vi "Set Window Position.vi"(7 "Module type":T1, 8 "error in (no error)":errorcluster, 11 "Vi reference":refnum<vi>) -> (0 "error out":errorcluster)   [LabVIEW 2021, in "Panther Dashboard.lvlib"]
uses:
  Panther Dashboard.lvlib
  Window Position--enum.ctl
  <vilib>/Utility/miscctls.llb/LVPointTypeDef.ctl
  <vilib>/Utility/miscctls.llb/LVRectTypeDef.ctl
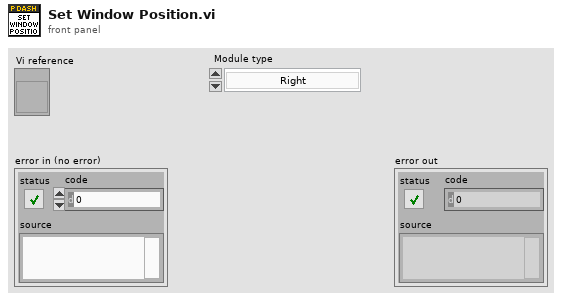
[diagram p1: front panel]
types:
  T1 = typedef "Panther Dashboard.lvlib/Window Position--enum.ctl" = enum16{"Right", "Left", "Center", "Max"}
  T2 = typedef "LVRectTypeDef.ctl" = cluster{"Left":i16, "Top":i16, "Right":i16, "Bottom":i16}
  T3 = typedef "LVPointTypeDef.ctl" = cluster{"Horizontal":i16, "Vertical":i16}
  T4 = enum32{"Invalid", "Standard", "Closed", "Hidden", "Minimized", "Maximized"}
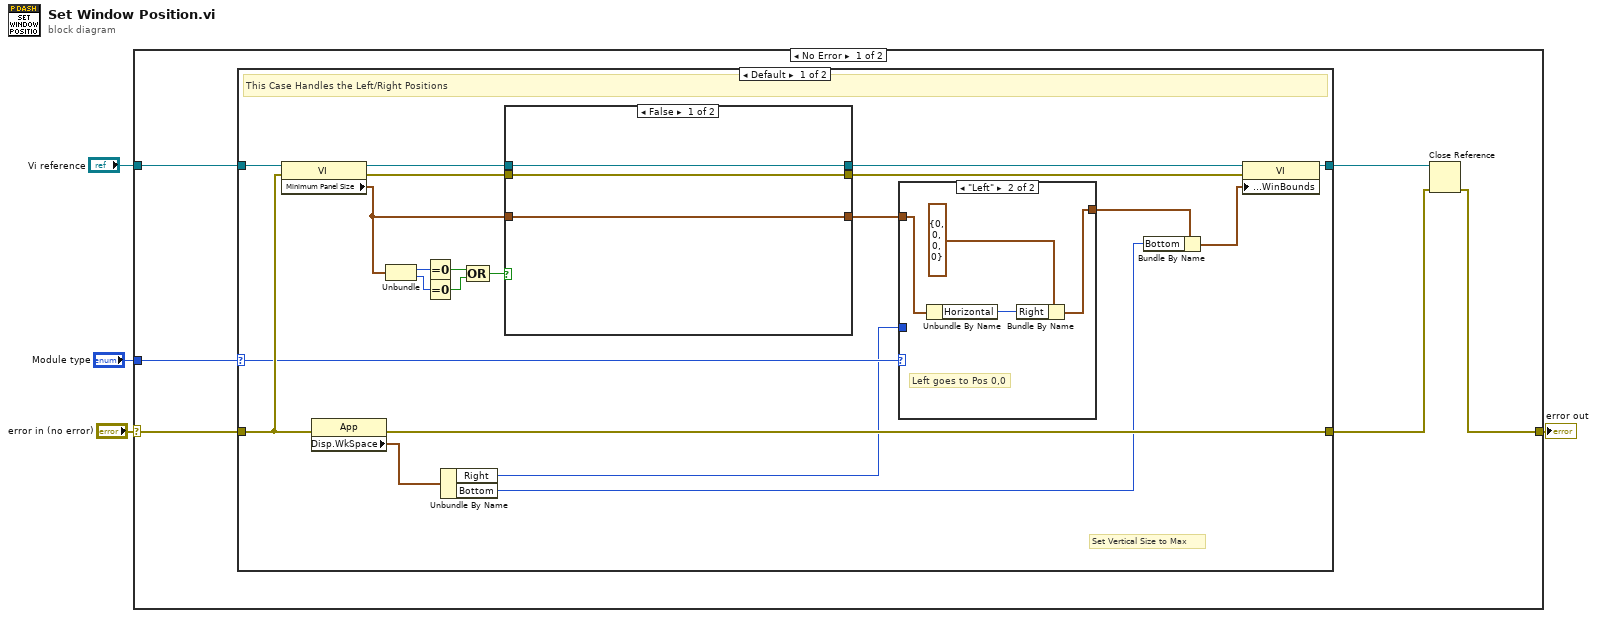
[diagram p0: block diagram]
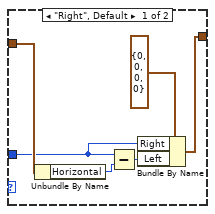
[diagram p2: hidden frame]
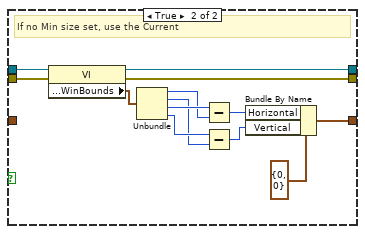
[diagram p3: hidden frame]
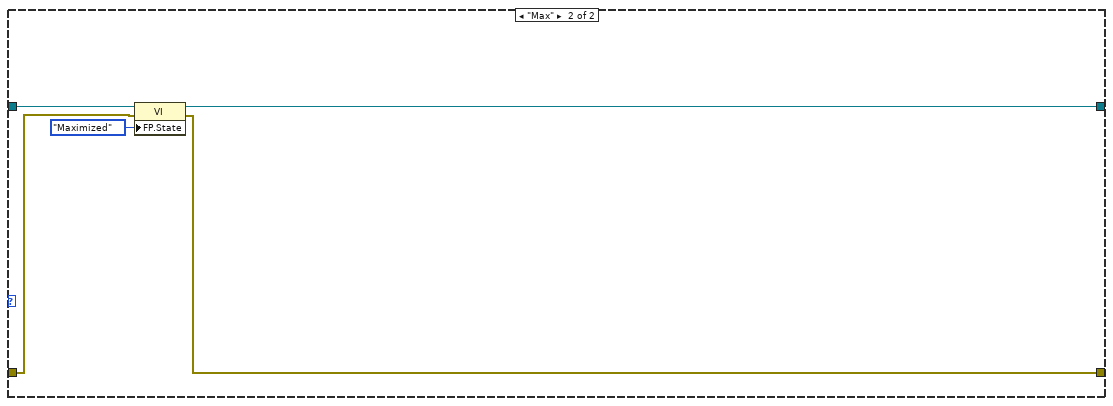
[diagram p4: hidden frame]
diagram:
  n1 = case shown="No Error" "error in (no error)" {
    selector: "error in (no error)" -> [w10 w63]
    tunnel: [w6 w63] -> w3
    tunnel: "Vi reference" -> [w5 _]
    tunnel: "Module type" -> [w9 _]
    frame No Error {
      n2 = case shown="Default" w9 {
        selector: w9 -> [w18 _]
        tunnel: [w31 w59] -> w7
        tunnel: w5 -> [w23 w61]
        tunnel: w10 -> [w21 w60]
        tunnel: [w14 w58] -> w8
        frame Default {
          # "Set Vertical Size to Max"
          # "This Case Handles the Left/Right Positions"
          n3 = property class="VI"(reference=w23, error in=w21) -> (reference out=w25:refnum<vi>, error out=w24:errorcluster, "Minimum Panel Size"=w22:T3)
          n4 = property class="App"(error in=w21) -> (error out=w31:errorcluster, "Disp.WkSpace"=w20:T2)  [unwired: 1 in, 1 out]
          n5 = Unbundle(w22) -> ("Horizontal"=w30:i16, "Vertical"=w29:i16)
          n6 = Equal To 0?(x=w30) -> (x = 0?=w28:bool)
          n7 = Equal To 0?(x=w29) -> (x = 0?=w27:bool)
          n8 = Unbundle By Name(w20) -> ("Right"=w16:i16, "Bottom"=w19:i16)
          n9 = Compound Arithmetic op=OR(w28, w27) -> (w26:bool)
          n10 = case shown="False" w26 {
            tunnel: w25 -> [w43 w57]
            tunnel: w24 -> [w42 w56]
            tunnel: [w44 w47] -> w17
            tunnel: w22 -> [w44 _]
            tunnel: [w42 w46] -> w13
            tunnel: [w43 w45] -> w15
            frame False {
            }
            frame True {
              # "If no Min size set, use the Current"
              n11 = property class="VI"(reference=w57, error in=w56) -> (reference out=w45:refnum<vi>, error out=w46:errorcluster, "Front Panel.WinBounds"=w55:T2)
              n12 = Unbundle(w55) -> ("Left"=w53:i16, "Top"=w51:i16, "Right"=w54:i16, "Bottom"=w52:i16)
              n13 = Subtract(x=w54, y=w53) -> (x-y=w50:i16)
              n14 = Subtract(x=w52, y=w51) -> (x-y=w48:i16)
              n15 = Bundle By Name(cluster=T3 {"Horizontal"=0, "Vertical"=0} ("Front Panel Window:Minimum Size"), "Horizontal"=w50, "Vertical"=w48) -> (w47:T3)
            }
          }
          n16 = case shown="\"Left\"" w18 {
            tunnel: w17 -> [w37 w39]
            tunnel: w16 -> [w32 _]
            tunnel: [w33 w40] -> w11
            frame "Right", Default {
              n17 = Unbundle By Name(w37) -> ("Horizontal"=w36:i16)
              n18 = Subtract(x=w32, y=w36) -> (x-y=w35:i16)
              n19 = Bundle By Name(cluster=T2 {"Left"=0, "Top"=0, "Right"=0, "Bottom"=0} ("Front Panel Window:Window Bounds"), "Right"=w32, "Left"=w35) -> (w33:T2)
            }
            frame "Left" {
              # "Left goes to Pos 0,0"
              n20 = Unbundle By Name(w39) -> ("Horizontal"=w38:i16)
              n21 = Bundle By Name(cluster=T2 {"Left"=0, "Top"=0, "Right"=0, "Bottom"=0} ("Front Panel Window:Window Bounds"), "Right"=w38) -> (w40:T2)
            }
          }
          n22 = Bundle By Name(cluster=w11, "Bottom"=w19) -> (w12:T2)
          n23 = property class="VI"(reference=w15, error in=w13, "Front Panel.WinBounds"=w12) -> (reference out=w14:refnum<vi>)  [unwired: 1 out]
        }
        frame "Max" {
          n24 = property class="VI"(reference=w61, error in=w60, "FP.State"=T4."Maximized" ("Front Panel Window:State")) -> (reference out=w58:refnum<vi>, error out=w59:errorcluster)
        }
      }
      n25 = Close Reference(reference=w8, error in (no error)=w7) -> (error out=w6:errorcluster)
    }
    frame Error {
    }
  }
  "error out" <- w3
